vi "SwissSPAD Live_Init FPGA v2.vi"(6 "Live Mode":bool, 8 "Error In":errorcluster, 11 "SwissSPAD Live Internal Variables in":T1={"okCFrontPanelDevices Refnum"=refnum, "Bottom Device Refnum"=refnum, "Display Image"=refnum, "# Live Images"=0, "relative s"=0.0, "# Image Sets"=0, "Message"="", "Current Image Set"=0, "# Datasets in Series"=0, "Current Dataset"=0, "Live Mode"=FALSE, "Recording Mode"=FALSE, "Record Button"=refnum, "\nLive Button"=refnum, "SwissSPAD Live Gate Image Data Q Name"="SS2 Live Gate Data Q", "Discard First Image"=FALSE, "Image Information"={"Save ROI Only"=FALSE, "Left"=0, "Top"=0, "Right"=0, "Bottom"=0, "Use Current ROI"=FALSE}, "Image Binning Options"={"Use Image Binning"=FALSE, "X Bin"=1, "Y Bin"=1}, "Bottom FPGA Serial Number"="", "Detector PCB Version"=enum."SS2 PCB1", "# Acquisitions"=1, "10 bits"=FALSE, "Top FPGA Serial Number"="", "Top Device Refnum"=refnum} {"# Acquisitions" min=1; "Image Binning Options"."Y Bin" min=1; "Image Binning Options"."X Bin" min=1}) -> (0 "Error Out":errorcluster, 1 "# 8-bit Images per Set":u32, 2 "Buffer Size (# 8-bit Images)":u32, 3 "SwissSPAD Live Internal Variables out":T1={"okCFrontPanelDevices Refnum"=refnum, "Bottom Device Refnum"=refnum, "Display Image"=refnum, "# Live Images"=0, "relative s"=0.0, "# Image Sets"=0, "Message"="", "Current Image Set"=0, "# Datasets in Series"=0, "Current Dataset"=0, "Live Mode"=FALSE, "Recording Mode"=FALSE, "Record Button"=refnum, "\nLive Button"=refnum, "SwissSPAD Live Gate Image Data Q Name"="SS2 Live Gate Data Q", "Discard First Image"=FALSE, "Image Information"={"Save ROI Only"=FALSE, "Left"=0, "Top"=0, "Right"=0, "Bottom"=0, "Use Current ROI"=FALSE}, "Image Binning Options"={"Use Image Binning"=FALSE, "X Bin"=1, "Y Bin"=1}, "Bottom FPGA Serial Number"="", "Detector PCB Version"=enum."SS2 PCB1", "# Acquisitions"=1, "10 bits"=FALSE, "Top FPGA Serial Number"="", "Top Device Refnum"=refnum} {"# Acquisitions" min=1; "Image Binning Options"."Y Bin" min=1; "Image Binning Options"."X Bin" min=1})   [LabVIEW 2021]
uses:
  SwissSPAD Live_Internal Variables.ctl
  D:/UCLA Thinkpad Google Drive/LabVIEW 2021 SP1/builds/SwissSPAD Live Distribution/Opal Kelly/C# Wrapper/v5.0.2/libFrontPanel-csharp.dll
  Opal Kelly/C# Wrapper/v5.0.2/libFrontPanel-csharp.dll
  <vilib>/vision/Image Controls.llb/IMAQ Image.ctl
  SwissSPAD Live_Image ROI Information.ctl
  Phasor/Image Binning Options.ctl
  SwissSPAD Live_SSx PCB Version.ctl
  SwissSPAD Live_Settings List.ctl
  Opal Kelly/C# Wrapper/okFrontPanelC#Wrapper.lvlib
  Variant/Variant to Data/Variant to Data.lvlib
panel:
  in  "milliseconds to wait":u32
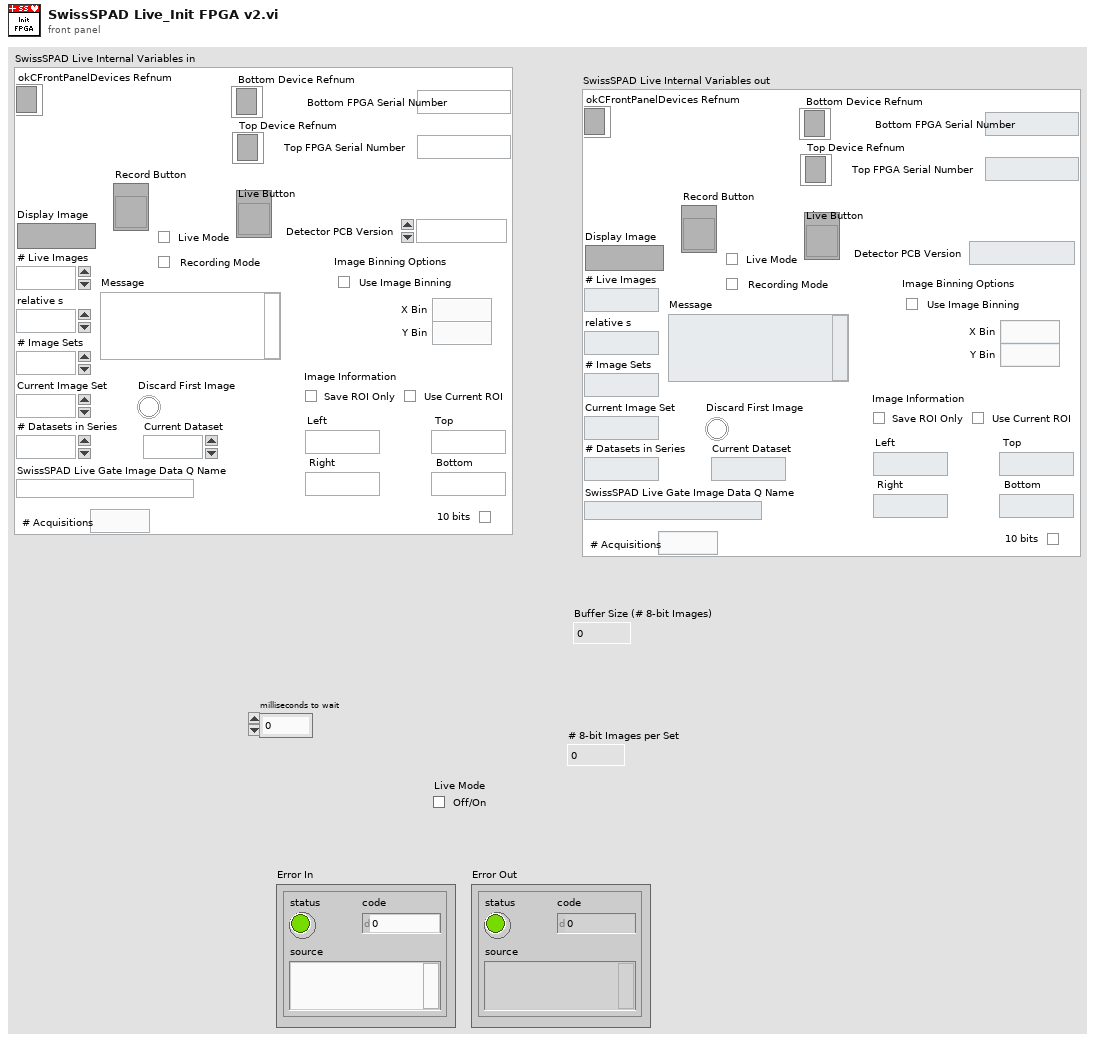
[diagram p1: front panel]
types:
  T1 = typedef "SwissSPAD Live_Internal Variables.ctl" = cluster{"okCFrontPanelDevices Refnum":refnum<k24>, "Bottom Device Refnum":refnum<k24>, "Display Image":T2, "# Live Images":i32, "relative s":dbl, "# Image Sets":i32, "Message":string, "Current Image Set":i32, "# Datasets in Series":i32, "Current Dataset":i32, "Live Mode":bool, "Recording Mode":bool, "Record Button":refnum<vi>, "\nLive Button":refnum<vi>, "SwissSPAD Live Gate Image Data Q Name":string, "Discard First Image":bool, "Image Information":T3, "Image Binning Options":T4, "Bottom FPGA Serial Number":string, "Detector PCB Version":T5, "# Acquisitions":u32, "10 bits":bool, "Top FPGA Serial Number":string, "Top Device Refnum":refnum<k24>}
  T2 = typedef "IMAQ Image.ctl" = refnum<image>
  T3 = typedef "SwissSPAD Live_Image ROI Information.ctl" = cluster{"Save ROI Only":bool, "Left":u16, "Top":u16, "Right":u16, "Bottom":u16, "Use Current ROI":bool}
  T4 = typedef "Image Binning Options.ctl" = cluster{"Use Image Binning":bool, "X Bin":i32, "Y Bin":i32}
  T5 = typedef "SwissSPAD Live_SSx PCB Version.ctl" = enum16{"unknown", "SS2 PCB1", "SS2 PCB2", "SS3 PCB1"}
  T6 = typedef "SwissSPAD Live_Settings List.ctl" = enum16{"FPGA:Bottom Half", "FPGA:Top Half", "FPGA:Bottom Bitfile Path", "FPGA:Top Bitfile Path", "FPGA:Bottom Bitstream Version", "FPGA:Top Bitstream Version", "FPGA:Auto Reset FPGA", "FPGA:Bottom FPGA Serial Number", "FPGA:Top FPGA Serial Number", "FPGA:Detector PCB Version", "Acquisition Parameters:Microlens", "Acquisition Parameters:SS2 DAQ Parameters", "Acquisition Parameters:Gate Configuration Array", "Acquisition Parameters:SS3 DAQ Parameters", "Acquisition Parameters:Buffer Size (# 8-bit Gates)", "File Information:File Information", "File Information:# Datasets in Series", "File Information:Scrambled File Flag", "File Information:SS3 Gate Slip Correction", "File Information:SS3 Hot Pixel Mismatch Detection", "File Information:Delay between Datasets", "File Information:Save Sum of All Gates Preview", "Image Parameters:Image ROI Information", "Image Parameters:Image Binning Options", "Image Parameters:SS3 Displayed Image", "Image Parameters:Image Display Options", "Image Parameters:Use Histogram Cursors", "Image Parameter:FPGA Data to Display", "UI Settings:Histogram Bins Number", "UI Settings:Use Image Display Options", "UI Settings:Verbose Settings", "UI Settings:Verbose Saving"}
  T7 = typedef "SwissSPAD Live_SS2 DAQ Parameters 3.ctl" = cluster{"10 bits":bool, "# Exposure Sequences":u32, "# 1-bit Frame per Gate":u32, "Gate Shift":u32, "# Gates per Set":u32, "# Sets":u32, "Laser Period":dbl[unit], "Sync Period":dbl[unit], "Gate Offset":u32, "Auto-adjust Gate Offset":bool, "Gate Definition":T8, "Reversed Shift":bool}
  T8 = typedef "SwissSPAD Live_SS2 Gate Definition.ctl" = cluster{"gs_psincdec_0":u32, "gs_psincdec_1":u32, "gs_psincdec_2":u32, "gs_psincdec_3":u32, "gs_no_shift_adj_1":u32, "gs_no_shift_adj_2":u32, "gs_no_shift_adj_3":u32}
  T9 = typedef "SwissSPAD Live_SS3 DAQ Parameters.ctl" = cluster{"10 bits":bool, "# Exposure Sequences":u32, "# 1-bit Frame per Gate":u32, "Gate Shift":u32, "# Gate Pairs per Set":u32, "# Sets":u32, "Laser Period":dbl[unit], "Sync Period":dbl[unit], "Gate Offset":u32, "Auto-adjust Gate Offset":bool, "Gate Definition":T10, "Gate Width (ns)":dbl, "Reversed Shift":bool, "Intensity Mode":bool, "Gate Definition Mode":T11}
  T10 = typedef "SwissSPAD Live_SS3 Gate Definition.ctl" = cluster{"gs_psincdec_0":u32, "gs_psincdec_1":u32, "gs_no_shift_adj_1":u32, "gate_adj_2":u32}
  T11 = typedef "SS3 Gate Width Definition Mode.ctl" = enum32{"Item 0", "Item 1"}
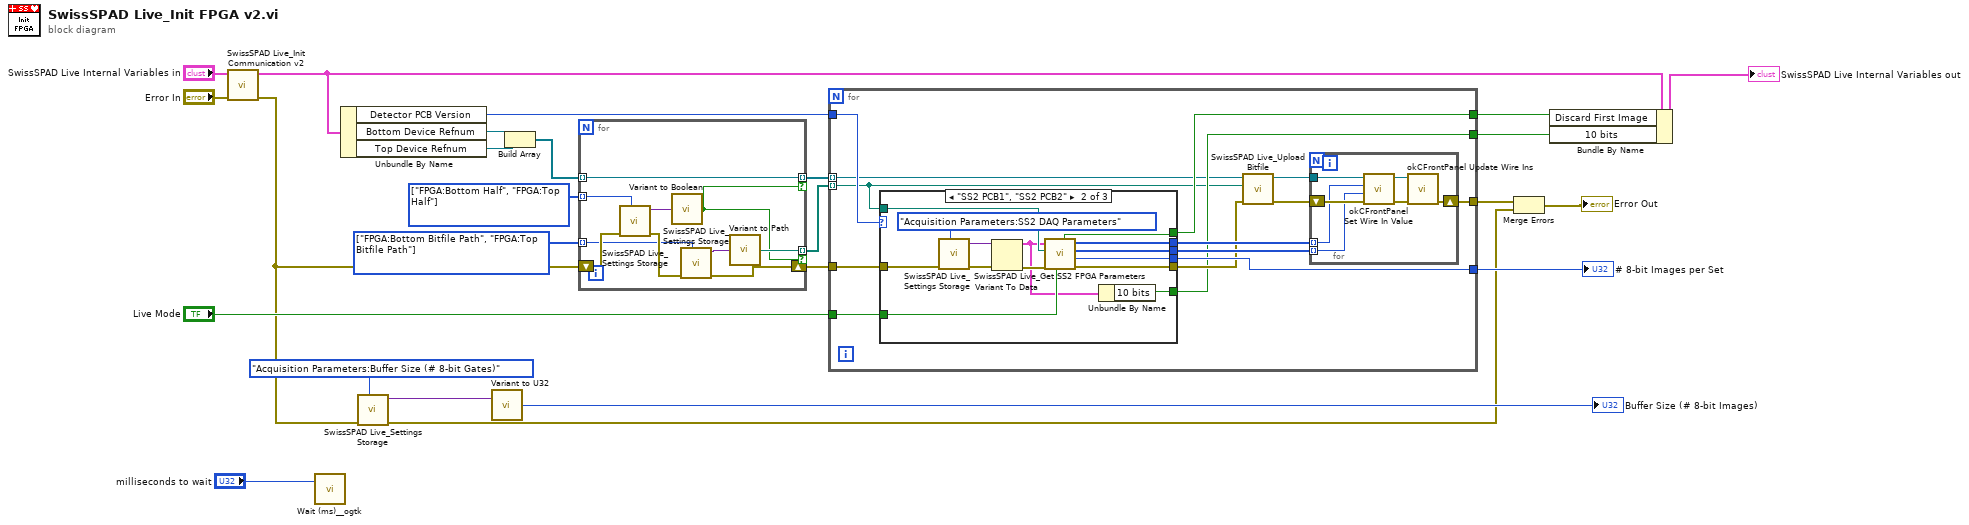
[diagram p0: block diagram]
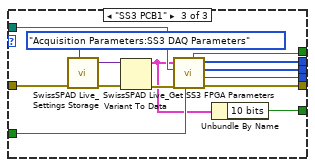
[diagram p3: hidden frame]
diagram:
  w13 = T6[] [enum."FPGA:Bottom Bitfile Path", enum."FPGA:Top Bitfile Path"] items=["FPGA:Bottom Half", "FPGA:Top Half", "FPGA:Bottom Bitfile Path", "FPGA:Top Bitfile Path", "FPGA:Bottom Bitstream Version", "FPGA:Top Bitstream Version", "FPGA:Auto Reset FPGA", "FPGA:Bottom FPGA Serial Number", "FPGA:Top FPGA Serial Number", "FPGA:Detector PCB Version", "Acquisition Parameters:Microlens", "Acquisition Parameters:SS2 DAQ Parameters", "Acquisition Parameters:Gate Configuration Array", "Acquisition Parameters:SS3 DAQ Parameters", "Acquisition Parameters:Buffer Size (# 8-bit Gates)", "File Information:File Information", "File Information:# Datasets in Series", "File Information:Scrambled File Flag", "File Information:SS3 Gate Slip Correction", "File Information:SS3 Hot Pixel Mismatch Detection", "File Information:Delay between Datasets", "File Information:Save Sum of All Gates Preview", "Image Parameters:Image ROI Information", "Image Parameters:Image Binning Options", "Image Parameters:SS3 Displayed Image", "Image Parameters:Image Display Options", "Image Parameters:Use Histogram Cursors", "Image Parameter:FPGA Data to Display", "UI Settings:Histogram Bins Number", "UI Settings:Use Image Display Options", "UI Settings:Verbose Settings", "UI Settings:Verbose Saving"] ("Array")
  w14 = T6[] [enum."FPGA:Bottom Half", enum."FPGA:Top Half"] items=["FPGA:Bottom Half", "FPGA:Top Half", "FPGA:Bottom Bitfile Path", "FPGA:Top Bitfile Path", "FPGA:Bottom Bitstream Version", "FPGA:Top Bitstream Version", "FPGA:Auto Reset FPGA", "FPGA:Bottom FPGA Serial Number", "FPGA:Top FPGA Serial Number", "FPGA:Detector PCB Version", "Acquisition Parameters:Microlens", "Acquisition Parameters:SS2 DAQ Parameters", "Acquisition Parameters:Gate Configuration Array", "Acquisition Parameters:SS3 DAQ Parameters", "Acquisition Parameters:Buffer Size (# 8-bit Gates)", "File Information:File Information", "File Information:# Datasets in Series", "File Information:Scrambled File Flag", "File Information:SS3 Gate Slip Correction", "File Information:SS3 Hot Pixel Mismatch Detection", "File Information:Delay between Datasets", "File Information:Save Sum of All Gates Preview", "Image Parameters:Image ROI Information", "Image Parameters:Image Binning Options", "Image Parameters:SS3 Displayed Image", "Image Parameters:Image Display Options", "Image Parameters:Use Histogram Cursors", "Image Parameter:FPGA Data to Display", "UI Settings:Histogram Bins Number", "UI Settings:Use Image Display Options", "UI Settings:Verbose Settings", "UI Settings:Verbose Saving"] ("Array")
  n1 = call "SwissSPAD Live_Init Communication v2.vi"("Error In"="Error In", "SwissSPAD Live Internal Variables in"="SwissSPAD Live Internal Variables in") -> ("Error Out"=w7:errorcluster, "SwissSPAD Live Internal Variables out"=w17:T1)  [unwired: 7 in, 1 out]
  n2 = call <userlib>:"Wait (ms)__ogtk.vi"("milliseconds to wait"="milliseconds to wait") -> ()  [unwired: 9 in, 2 out]
  n3 = Unbundle By Name(w17) -> ("Detector PCB Version"=w16:T5, "Bottom Device Refnum"=w12:refnum<k24>, "Top Device Refnum"=w11:refnum<k24>)
  n4 = call "SwissSPAD Live_Settings Storage.vi"("Settings List"=SwissSPAD_Live_Settings_List."Acquisition Parameters:Buffer Size (# 8-bit Gates)", "Error In"=w7) -> ("Error Out"=w4:errorcluster, "Variant Data out"=w1:variant)  [unwired: 8 in]
  n5 = call "Variant to U32.vi"("Variant"=w1) -> ("Value"=→"Buffer Size (# 8-bit Images)":u32)  [unwired: 8 in]
  n6 = Build Array(w12, w11) -> (w10:refnum<k24>[])
  n7 = for {
    tunnel: w14 -> [w29] mode=indexing
    tunnel: w13 -> [w27] mode=indexing
    tunnel: [w34] -> w8 mode=indexing if=w33
    tunnel: w10 -> [w31] mode=indexing
    tunnel: [w31] -> w9 mode=indexing if=w33
    shift-right: [w32] -> w3
    shift-left: w7 -> [w30]
    n8 = call "SwissSPAD Live_Settings Storage.vi"("Settings List"=w29, "Error In"=w30) -> ("Error Out"=w35:errorcluster, "Variant Data out"=w28:variant)  [unwired: 8 in]
    n9 = call "Variant to Boolean.vi"("Variant"=w28) -> ("Value"=w33:bool)  [unwired: 8 in]
    n10 = call "SwissSPAD Live_Settings Storage.vi"("Settings List"=w27, "Error In"=w35) -> ("Error Out"=w32:errorcluster, "Variant Data out"=w26:variant)  [unwired: 8 in]
    n11 = call "Variant to Path.vi"("Variant"=w26) -> ("Path"=w34:path)  [unwired: 8 in]
  }
  n12 = for {
    tunnel: [w47] -> w6
    tunnel: [w44] -> w24
    tunnel: w16 -> [w40]
    tunnel: [w39] -> w15
    tunnel: "Live Mode" -> [w43]
    tunnel: [w42] -> w19
    tunnel: w9 -> [w38] mode=indexing
    tunnel: w8 -> [w37] mode=indexing
    tunnel: w3 -> [w36]
    n13 = case shown="\"SS2 PCB1\", \"SS2 PCB2\"" w40 {
      tunnel: [_ w64 w78] -> w46
      tunnel: [_ w63 w77] -> w45
      tunnel: [_ w60 w74] -> w44
      tunnel: w43 -> [_ w59 w73]
      tunnel: w37 -> [_ w58 w72]
      tunnel: w36 -> [w50 w55 w71]
      tunnel: [_ w57 w70] -> w42
      tunnel: [w50 w56 w69] -> w41
      tunnel: [_ w53 w67] -> w39
      frame "unknown", Default {
      }
      frame "SS2 PCB1", "SS2 PCB2" {
        n14 = call "SwissSPAD Live_Settings Storage.vi"("Settings List"=SwissSPAD_Live_Settings_List."Acquisition Parameters:SS2 DAQ Parameters", "Error In"=w55) -> ("Error Out"=w62:errorcluster, "Variant Data out"=w51:variant)  [unwired: 8 in]
        n15 = Variant To Data(error in=w62, Variant=w51) -> (data=w54:T7, error out=w61:errorcluster)  [unwired: 1 in]
        n16 = call "SwissSPAD Live_Get SS2 FPGA Parameters.vi"("Live Mode"=w59, "Error In"=w61, "Bifile Path"=w58, "SS2 DAQ Parameters"=w54) -> ("Error Out"=w56:errorcluster, "#8-bit Images per Set"=w60:u32, "SS2 FPGA DAQ Parameters"=w64:u32[], "SS2 FPGA DAQ Addresses"=w63:i32[], "Discard First Image"=w57:bool)  [unwired: 3 in]
        n17 = Unbundle By Name(w54) -> ("10 bits"=w53:bool)
      }
      frame "SS3 PCB1" {
        n18 = call "SwissSPAD Live_Settings Storage.vi"("Settings List"=SwissSPAD_Live_Settings_List."Acquisition Parameters:SS3 DAQ Parameters", "Error In"=w71) -> ("Error Out"=w76:errorcluster, "Variant Data out"=w65:variant)  [unwired: 8 in]
        n19 = Variant To Data(error in=w76, Variant=w65) -> (data=w68:T9, error out=w75:errorcluster)  [unwired: 1 in]
        n20 = call "SwissSPAD Live_Get SS3 FPGA Parameters.vi"("Live Mode"=w73, "Error In"=w75, "Bifile Path"=w72, "SS3 DAQ Parameters"=w68) -> ("Error Out"=w69:errorcluster, "# 8-bit Images per Set"=w74:u32, "SS3 FPGA DAQ Parameters"=w78:u32[], "SS3 FPGA DAQ Addresses"=w77:i32[], "Discard First Image"=w70:bool)  [unwired: 3 in]
        n21 = Unbundle By Name(w68) -> ("10 bits"=w67:bool)
      }
    }
    n22 = call "SwissSPAD Live_Upload Bitfile.vi"("error in (no error)"=w41, "FPGA bitfile Path"=w37, "okCFrontPanel Device Refnum"=w38) -> ("error out"=w49:errorcluster, "okCFrontPanel Device Refnum"=w48:refnum<k24>)  [unwired: 7 in]
    n23 = for {
      shift-right: [w80] -> w47
      shift-left: w49 -> [w85]
      tunnel: w46 -> [w83] mode=indexing
      tunnel: w45 -> [w79] mode=indexing
      tunnel: w48 -> [w84]
      n24 = call "okCFrontPanel Set Wire In Value.vi"("Error In"=w85, "Value"=w83, "Endpoint"=w79, "okCFrontPanel Refnum"=w84) -> ("Error Out"=w82:errorcluster, "okCFrontPanel Refnum"=w81:refnum<k24>)  [unwired: 6 in]
      n25 = call "okCFrontPanel Update Wire Ins.vi"("Error In"=w82, "okCFrontPanel Refnum"=w81) -> ("Error Out"=w80:errorcluster)  [unwired: 8 in, 1 out]
    }
  }
  "# 8-bit Images per Set" <- w24
  n26 = Merge Errors(w6, w4) -> (→"Error Out":errorcluster)
  n27 = Bundle By Name(cluster=w17, "Discard First Image"=w19, "10 bits"=w15) -> (→"SwissSPAD Live Internal Variables out":T1)
